vi "Write Pot Value.vi"   [LabVIEW 2012]
uses:
  <vilib>/Rock Robotics/WPI/Joystick/WPI_JoystickGetSetRefNum.vi
types:
  T1 = typedef "WPI_AnalogChannelDevRef.ctl" = cluster{"DevStatus":errorcluster, "Analog Module":T2, "Analog Channel":T3}
  T2 = typedef "FPGA_TypedefAnalogModule.ctl" = enum16{"Analog Module 1", "Analog Module 2"}
  T3 = typedef "FPGA_AIChannel.ctl" = enum8{"AI 1", "AI 2", "AI 3", "AI 4", "AI 5", "AI 6", "AI 7", "AI 8", "Invalid"}
  T4 = typedef "WPI_JoystickDevRef.ctl" = cluster{"Device":T5}
  T5 = typedef "WPI_JoystickDeviceEnum.ctl" = enum16{"USB 1", "USB 2", "USB 3", "USB 4", "Kinect 1", "Kinect 2"}
  T6 = typedef "WPI_JoystickButtonState.ctl" = cluster{"Button 1":bool, "Button 2":bool, "Button 3":bool, "Button 4":bool, "Button 5":bool, "Button 6":bool, "Button 7":bool, "Button 8":bool, "Button 9":bool, "Button 10":bool, "Button 11":bool, "Button 12":bool}
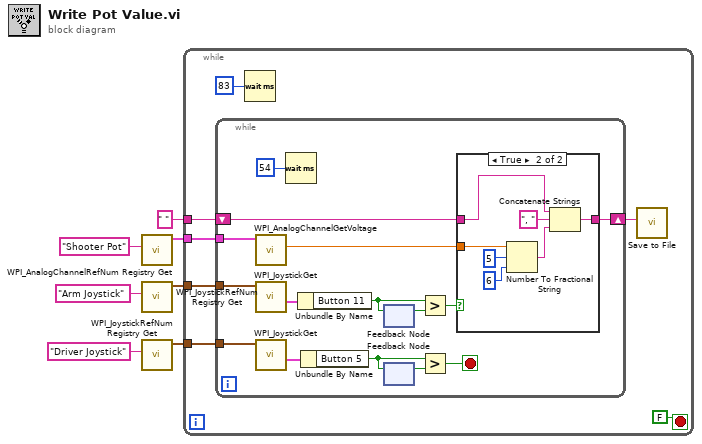
[diagram p0: block diagram]
diagram:
  n1 = call <vilib>:"WPI_AnalogChannelRefNum Registry Get.vi"("refnum name"="Shooter Pot") -> ("AIDeviceRef"=w3:T1)  [unwired: 9 in, 1 out]
  n2 = call <vilib>:"WPI_JoystickRefNum Registry Get.vi"("refnum name"="Arm Joystick") -> ("JoystickDevRef"=w2:T4)  [unwired: 9 in, 1 out]
  n3 = call <vilib>:"WPI_JoystickRefNum Registry Get.vi"("refnum name"="Driver Joystick") -> ("JoystickDevRef"=w1:T4)  [unwired: 9 in, 1 out]
  n4 = while {
    tunnel: " " ("string") -> [w14]
    tunnel: w3 -> [w13]
    tunnel: w2 -> [w12]
    tunnel: w1 -> [w11]
    stop <- FALSE stop-if-true
    n5 = while {
      shift-right: [w18] -> w8
      shift-left: w14 -> [w28]
      tunnel: w12 -> [w25]
      tunnel: w13 -> [w22]
      tunnel: w11 -> [w20]
      stop <- w15 stop-if-true
      n6 = call <vilib>:"WPI_AnalogChannelGetVoltage.vi"("AIDeviceRef"=w22) -> ("Voltage"=w21:dbl)  [unwired: 8 in, 2 out]
      n7 = call <vilib>:"WPI_JoystickGet.vi"("JoystickDevRef"=w25) -> ("Buttons"=w24:T6)  [unwired: 4 in, 2 out]
      n8 = call <vilib>:"WPI_JoystickGet.vi"("JoystickDevRef"=w20) -> ("Buttons"=w19:T6)  [unwired: 4 in, 2 out]
      n9 = Wait (ms)(milliseconds to wait=u32 54) -> ()  [unwired: 1 out]
      n10 = Unbundle By Name(w24) -> ("Button 11"=w23:bool)
      n11 = Unbundle By Name(w19) -> ("Button 5"=w16:bool)
      n12 = feedback-in #1(w23) -> ()
      n13 = feedback #1() -> (w27:bool)  [unwired: 1 in]
      n14 = feedback #2() -> (w17:bool)  [unwired: 1 in]
      n15 = feedback-in #2(w16) -> ()
      n16 = Greater?(x=w23, y=w27) -> (0:w26:bool)
      n17 = Greater?(x=w16, y=w17) -> (0:w15:bool)
      n18 = case shown="True" w26 {
        tunnel: w28 -> [w30 w34]
        tunnel: [w30 w33] -> w18
        tunnel: w21 -> [_ w32]
        frame False {
        }
        frame True {
          n19 = Number To Fractional String(number=w32, width (-)=i16 5, precision (6)=i16 6) -> (F-format string=w35:string)  [unwired: 1 in]
          n20 = Concatenate Strings(w34, ", " ("string"), w35) -> (w33:string)
        }
      }
    }
    n21 = Wait (ms)(milliseconds to wait=u32 83) -> ()  [unwired: 1 out]
    n22 = call "Save to File.vi"("Text in"=w8) -> ()  [unwired: 11 in]
  }
